vi "GetMIDASConnectionStatus.vi"() -> (1 "Seconds since last communication with MIDAS":dbl, 3 "MIDAS Connection OK":bool)   [LabVIEW 2018, in "feGEM DataPacker.lvlib"]
uses:
  feGEM DataPacker.lvlib
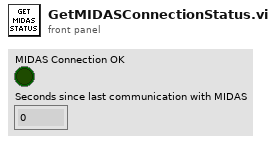
[diagram p1: front panel]
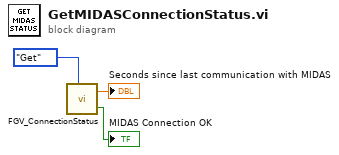
[diagram p0: block diagram]
diagram:
  n1 = call "FGV_ConnectionStatus.vi"("Enum"=enum16{"Get", "Set"}."Get") -> ("Seconds since last communication with MIDAS"=→"Seconds since last communication with MIDAS":dbl, "MIDAS Connection OK"=→"MIDAS Connection OK":bool)  [unwired: 4 in]
